vi "WinchPositionControl.vi"(11 "Buttons":bool[](array[boolean])=[FALSE, FALSE, FALSE, FALSE, FALSE, FALSE, FALSE, FALSE, FALSE, FALSE, FALSE, FALSE]) -> ()   [LabVIEW 2015]
uses:
  <vilib>/Rock Robotics/WPI/Utilities/WPI_GetSetVariantRefNum.vi
  Utilities/MotorPositionGlobals.vi
panel:
  in  "t 2":dbl=5400.0 format="%#_13g"
  in  "t":dbl=2325.0 format="%#_13g"
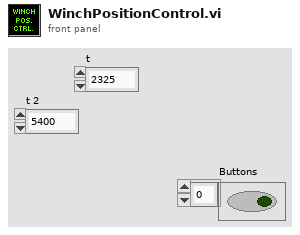
[diagram p1: front panel]
types:
  T1 = typedef "WPI_JoystickDevRef.ctl" = cluster{"Device":T2}
  T2 = typedef "WPI_JoystickDeviceEnum.ctl" = enum16{"USB 0", "USB 1", "USB 2", "USB 3", "USB 4", "USB 5"}
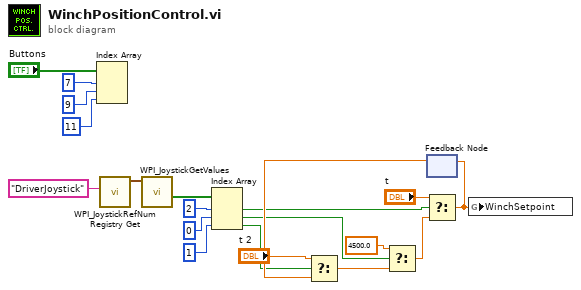
[diagram p0: block diagram]
diagram:
  n1 = Index Array(array="Buttons", index #1=7 ("index"), index #2=9 ("index"), index #3=11 ("index")) -> ()  [unwired: 3 out]
  n2 = call <vilib>:"WPI_JoystickRefNum Registry Get.vi"("refnum name"="DriverJoystick") -> ("JoystickDevRef"=w8:T1)  [unwired: 9 in, 1 out]
  n3 = call <vilib>:"WPI_JoystickGetValues.vi"("JoystickDevRef"=w8) -> ("Buttons"=w7:bool[])  [unwired: 6 in, 4 out]
  n4 = Index Array(array=w7, index #1=2 ("index"), index #2=0 ("index"), index #3=1 ("index")) -> (element #1=w3:bool, element #2=w2:bool, element #3=w1:bool)
  n5 = feedback #1() -> (w10:dbl)  [unwired: 1 in]
  n6 = Select(t="t 2", s=w1, f=w10) -> (s? t:f=w20:dbl)
  n7 = Select(t=4500.0, s=w2, f=w20) -> (s? t:f=w19:dbl)
  n8 = Select(t="t", s=w3, f=w19) -> (s? t:f=w11:dbl)
  n9 = feedback-in #1(w11) -> ()
  n10 = global write "MotorPositionGlobals.vi" "WinchSetpoint"(w11) -> ()
